vi "GeoData.vi"() -> ()   [LabVIEW 2017] (continued)
29826\t45011\tElko\tSC\tBarnwell County\tH1\n29915\t45013\tDaufuskie island\tSC\tBeaufort County\tH1\n29907\t45013\tBeaufort\tSC\tBeaufort County\tH1\n29910\t45013\tBluffton\tSC\tBeaufort County\tH1\n29909\t45013\tOkatie\tSC\tBeaufort County\tH1\n29906\t45013\tBeaufort\tSC\tBeaufort County\tH1\n29920\t45013\tSaint helena island\tSC\tBeaufort County\tH1\n29925\t45013\tHilton head island\tSC\tBeaufort County\tH1\n29936\t45013\tRidgeland\tSC\tBeaufort County\tH1\n29935\t45013\tPort royal\tSC\tBeaufort County\tH1\n29904\t45013\tBeaufort\tSC\tBeaufort County\tH1\n29926\t45013\tHilton head island\tSC\tBeaufort County\tH1\n29940\t45013\tSeabrook\tSC\tBeaufort County\tH1\n29945\t45013\tYemassee\tSC\tBeaufort County\tH1\n29902\t45013\tBeaufort\tSC\tBeaufort County\tH1\n29903\t45013\tBeaufort\tSC\tBeaufort County\tH1\n29901\t45013\tBeaufort\tSC\tBeaufort County\tH1\n29931\t45013\tLobeco\tSC\tBeaufort County\tH1\n29905\t45013\tParris island\tSC\tBeaufort County\tH1\n29928\t45013\tHilton head island\tSC\tBeaufort County\tH1\n29938\t45013\tHilton head island\tSC\tBeaufort County\tH1\n29941\t45013\tSheldon\tSC\tBeaufort County\tH1\n29431\t45015\tBonneau\tSC\tBerkeley County\tH1\n29456\t45015\tLadson\tSC\tBerkeley County\tH1\n29461\t45015\tMoncks corner\tSC\tBerkeley County\tH1\n29466\t45015\tMount pleasant\tSC\tBerkeley County\tH1\n29469\t45015\tPinopolis\tSC\tBerkeley County\tH1\n29059\t45015\tHolly hill\tSC\tBerkeley County\tH1\n29472\t45015\tRidgeville\tSC\tBerkeley County\tH1\n29406\t45015\tCharleston\tSC\tBerkeley County\tH1\n29492\t45015\tCharleston\tSC\tBerkeley County\tH1\n29453\t45015\tJamestown\tSC\tBerkeley County\tH1\n29445\t45015\tGoose creek\tSC\tBerkeley County\tH1\n29468\t45015\tPineville\tSC\tBerkeley County\tH1\n29450\t45015\tHuger\tSC\tBerkeley County\tH1\n29410\t45015\tHanahan\tSC\tBerkeley County\tH1\n29483\t45015\tSummerville\tSC\tBerkeley County\tH1\n29436\t45015\tCross\tSC\tBerkeley County\tH1\n29486\t45015\tSummerville\tSC\tBerkeley County\tH1\n29434\t45015\tCordesville\tSC\tBerkeley County\tH1\n29479\t45015\tSaint stephen\tSC\tBerkeley County\tH1\n29476\t45015\tRussellville\tSC\tBerkeley County\tH1\n29118\t45017\tOrangeburg\tSC\tCalhoun County\tH1\n29053\t45017\tGaston\tSC\tCalhoun County\tH1\n29135\t45017\tSaint matthews\tSC\tCalhoun County\tH1\n29030\t45017\tCameron\tSC\tCalhoun County\tH1\n29047\t45017\tElloree\tSC\tCalhoun County\tH1\n29160\t45017\tSwansea\tSC\tCalhoun County\tH1\n29112\t45017\tNorth\tSC\tCalhoun County\tH1\n29455\t45019\tJohns island\tSC\tCharleston County\tH1\n29449\t45019\tHollywood\tSC\tCharleston County\tH1\n29424\t45019\tCharleston\tSC\tCharleston County\tH1\n29456\t45019\tLadson\tSC\tCharleston County\tH1\n29466\t45019\tMount pleasant\tSC\tCharleston County\tH1\n29465\t45019\tMount pleasant\tSC\tCharleston County\tH1\n29417\t45019\tCharleston\tSC\tCharleston County\tH1\n29412\t45019\tCharleston\tSC\tCharleston County\tH1\n29401\t45019\tCharleston\tSC\tCharleston County\tH1\n29419\t45019\tNorth charleston\tSC\tCharleston County\tH1\n29413\t45019\tCharleston\tSC\tCharleston County\tH1\n29439\t45019\tFolly beach\tSC\tCharleston County\tH1\n29406\t45019\tCharleston\tSC\tCharleston County\tH1\n29438\t45019\tEdisto island\tSC\tCharleston County\tH1\n29429\t45019\tAwendaw\tSC\tCharleston County\tH1\n29464\t45019\tMount pleasant\tSC\tCharleston County\tH1\n29485\t45019\tSummerville\tSC\tCharleston County\tH1\n29470\t45019\tRavenel\tSC\tCharleston County\tH1\n29453\t45019\tJamestown\tSC\tCharleston County\tH1\n29409\t45019\tCharleston\tSC\tCharleston County\tH1\n29451\t45019\tIsle of palms\tSC\tCharleston County\tH1\n29450\t45019\tHuger\tSC\tCharleston County\tH1\n29482\t45019\tSullivans island\tSC\tCharleston County\tH1\n29416\t45019\tCharleston\tSC\tCharleston County\tH1\n29426\t45019\tAdams run\tSC\tCharleston County\tH1\n29403\t45019\tCharleston\tSC\tCharleston County\tH1\n29407\t45019\tCharleston\tSC\tCharleston County\tH1\n29405\t45019\tNorth charleston\tSC\tCharleston County\tH1\n29410\t45019\tHanahan\tSC\tCharleston County\tH1\n29422\t45019\tCharleston\tSC\tCharleston County\tH1\n29483\t45019\tSummerville\tSC\tCharleston County\tH1\n29415\t45019\tNorth charleston\tSC\tCharleston County\tH1\n29425\t45019\tCharleston\tSC\tCharleston County\tH1\n29404\t45019\tCharleston afb\tSC\tCharleston County\tH1\n29418\t45019\tNorth charleston\tSC\tCharleston County\tH1\n29420\t45019\tNorth charleston\tSC\tCharleston County\tH1\n29414\t45019\tCharleston\tSC\tCharleston County\tH1\n29487\t45019\tWadmalaw island\tSC\tCharleston County\tH1\n29423\t45019\tCharleston\tSC\tCharleston County\tH1\n29402\t45019\tCharleston\tSC\tCharleston County\tH1\n29458\t45019\tMc clellanville\tSC\tCharleston County\tH1\n29457\t45019\tJohns island\tSC\tCharleston County\tH1\n29702\t45021\tBlacksburg\tSC\tCherokee County\tH1\n29306\t45021\tSpartanburg\tSC\tCherokee County\tH1\n29323\t45021\tChesnee\tSC\tCherokee County\tH1\n29341\t45021\tGaffney\tSC\tCherokee County\tH1\n29330\t45021\tCowpens\tSC\tCherokee County\tH1\n29372\t45021\tPacolet\tSC\tCherokee County\tH1\n29340\t45021\tGaffney\tSC\tCherokee County\tH1\n29307\t45021\tSpartanburg\tSC\tCherokee County\tH1\n29743\t45021\tSmyrna\tSC\tCherokee County\tH1\n29714\t45023\tFort lawn\tSC\tChester County\tH1\n29031\t45023\tCarlisle\tSC\tChester County\tH1\n29742\t45023\tSharon\tSC\tChester County\tH1\n29706\t45023\tChester\tSC\tChester County\tH1\n29014\t45023\tBlackstock\tSC\tChester County\tH1\n29704\t45023\tCatawba\tSC\tChester County\tH1\n29730\t45023\tRock hill\tSC\tChester County\tH1\n29712\t45023\tEdgemoor\tSC\tChester County\tH1\n29729\t45023\tRichburg\tSC\tChester County\tH1\n29055\t45023\tGreat falls\tSC\tChester County\tH1\n29720\t45025\tLancaster\tSC\tChesterfield County\tH1\n29584\t45025\tPatrick\tSC\tChesterfield County\tH1\n29741\t45025\tRuby\tSC\tChesterfield County\tH1\n29520\t45025\tCheraw\tSC\tChesterfield County\tH1\n29727\t45025\tMount croghan\tSC\tChesterfield County\tH1\n29101\t45025\tMc bee\tSC\tChesterfield County\tH1\n29718\t45025\tJefferson\tSC\tChesterfield County\tH1\n29009\t45025\tBethune\tSC\tChesterfield County\tH1\n29550\t45025\tHartsville\tSC\tChesterfield County\tH1\n29593\t45025\tSociety hill\tSC\tChesterfield County\tH1\n29728\t45025\tPageland\tSC\tChesterfield County\tH1\n29709\t45025\tChesterfield\tSC\tChesterfield County\tH1\n29111\t45027\tNew zion\tSC\tClarendon County\tH1\n29056\t45027\tGreeleyville\tSC\tClarendon County\tH1\n29162\t45027\tTurbeville\tSC\tClarendon County\tH1\n29102\t45027\tManning\tSC\tClarendon County\tH1\n29148\t45027\tSummerton\tSC\tClarendon County\tH1\n29518\t45027\tCades\tSC\tClarendon County\tH1\n29041\t45027\tDavis station\tSC\tClarendon County\tH1\n29051\t45027\tGable\tSC\tClarendon County\tH1\n29114\t45027\tOlanta\tSC\tClarendon County\tH1\n29001\t45027\tAlcolu\tSC\tClarendon County\tH1\n29125\t45027\tPinewood\tSC\tClarendon County\tH1\n29560\t45027\tLake city\tSC\tClarendon County\tH1\n29474\t45029\tRound o\tSC\tColleton County\tH1\n29475\t45029\tRuffin\tSC\tColleton County\tH1\n29472\t45029\tRidgeville\tSC\tColleton County\tH1\n29438\t45029\tEdisto island\tSC\tColleton County\tH1\n29446\t45029\tGreen pond\tSC\tColleton County\tH1\n29945\t45029\tYemassee\tSC\tColleton County\tH1\n29081\t45029\tEhrhardt\tSC\tColleton County\tH1\n29481\t45029\tSmoaks\tSC\tColleton County\tH1\n29929\t45029\tIslandton\tSC\tColleton County\tH1\n29452\t45029\tJacksonboro\tSC\tColleton County\tH1\n29082\t45029\tLodge\tSC\tColleton County\tH1\n29435\t45029\tCottageville\tSC\tColleton County\tH1\n29432\t45029\tBranchville\tSC\tColleton County\tH1\n29488\t45029\tWalterboro\tSC\tColleton County\tH1\n29493\t45029\tWilliams\tSC\tColleton County\tH1\n29501\t45031\tFlorence\tSC\tDarlington County\tH1\n29540\t45031\tDarlington\tSC\tDarlington County\tH1\n29101\t45031\tMc bee\tSC\tDarlington County\tH1\n29551\t45031\tHartsville\tSC\tDarlington County\tH1\n29069\t45031\tLamar\tSC\tDarlington County\tH1\n29161\t45031\tTimmonsville\tSC\tDarlington County\tH1\n29550\t45031\tHartsville\tSC\tDarlington County\tH1\n29593\t45031\tSociety hill\tSC\tDarlington County\tH1\n29079\t45031\tLydia\tSC\tDarlington County\tH1\n29506\t45031\tFlorence\tSC\tDarlington County\tH1\n29532\t45031\tDarlington\tSC\tDarlington County\tH1\n29574\t45033\tMullins\tSC\tDillon County\tH1\n29536\t45033\tDillon\tSC\tDillon County\tH1\n29565\t45033\tLatta\tSC\tDillon County\tH1\n29567\t45033\tLittle rock\tSC\tDillon County\tH1\n29563\t45033\tLake view\tSC\tDillon County\tH1\n29581\t45033\tNichols\tSC\tDillon County\tH1\n29592\t45033\tSellers\tSC\tDillon County\tH1\n29547\t45033\tHamer\tSC\tDillon County\tH1\n29525\t45033\tClio\tSC\tDillon County\tH1\n29543\t45033\tFork\tSC\tDillon County\tH1\n29571\t45033\tMarion\tSC\tDillon County\tH1\n29437\t45035\tDorchester\tSC\tDorchester County\tH1\n29456\t45035\tLadson\tSC\tDorchester County\tH1\n29484\t45035\tSummerville\tSC\tDorchester County\tH1\n29472\t45035\tRidgeville\tSC\tDorchester County\tH1\n29471\t45035\tReevesville\tSC\tDorchester County\tH1\n29485\t45035\tSummerville\tSC\tDorchester County\tH1\n29470\t45035\tRavenel\tSC\tDorchester County\tH1\n29426\t45035\tAdams run\tSC\tDorchester County\tH1\n29483\t45035\tSummerville\tSC\tDorchester County\tH1\n29418\t45035\tNorth charleston\tSC\tDorchester County\tH1\n29420\t45035\tNorth charleston\tSC\tDorchester County\tH1\n29414\t45035\tCharleston\tSC\tDorchester County\tH1\n29432\t45035\tBranchville\tSC\tDorchester County\tH1\n29477\t45035\tSaint george\tSC\tDorchester County\tH1\n29447\t45035\tGrover\tSC\tDorchester County\tH1\n29018\t45035\tBowman\tSC\tDorchester County\tH1\n29448\t45035\tHarleyville\tSC\tDorchester County\tH1\n29841\t45037\tNorth augusta\tSC\tEdgefield County\tH1\n29129\t45037\tRidge spring\tSC\tEdgefield County\tH1\n29138\t45037\tSaluda\tSC\tEdgefield County\tH1\n29824\t45037\tEdgefield\tSC\tEdgefield County\tH1\n29838\t45037\tModoc\tSC\tEdgefield County\tH1\n29847\t45037\tTrenton\tSC\tEdgefield County\tH1\n29821\t45037\tClarks hill\tSC\tEdgefield County\tH1\n29860\t45037\tNorth augusta\tSC\tEdgefield County\tH1\n29835\t45037\tMc cormick\tSC\tEdgefield County\tH1\n29845\t45037\tPlum branch\tSC\tEdgefield County\tH1\n29832\t45037\tJohnston\tSC\tEdgefield County\tH1\n29065\t45039\tJenkinsville\tSC\tFairfield County\tH1\n29015\t45039\tBlair\tSC\tFairfield County\tH1\n29031\t45039\tCarlisle\tSC\tFairfield County\tH1\n29045\t45039\tElgin\tSC\tFairfield County\tH1\n29180\t45039\tWinnsboro\tSC\tFairfield County\tH1\n29014\t45039\tBlackstock\tSC\tFairfield County\tH1\n29016\t45039\tBlythewood\tSC\tFairfield County\tH1\n29132\t45039\tRion\tSC\tFairfield County\tH1\n29130\t45039\tRidgeway\tSC\tFairfield County\tH1\n29055\t45039\tGreat falls\tSC\tFairfield County\tH1\n29162\t45041\tTurbeville\tSC\tFlorence County\tH1\n29501\t45041\tFlorence\tSC\tFlorence County\tH1\n29541\t45041\tEffingham\tSC\tFlorence County\tH1\n29555\t45041\tJohnsonville\tSC\tFlorence County\tH1\n29502\t45041\tFlorence\tSC\tFlorence County\tH1\n29505\t45041\tFlorence\tSC\tFlorence County\tH1\n29554\t45041\tHemingway\tSC\tFlorence County\tH1\n29504\t45041\tFlorence\tSC\tFlorence County\tH1\n29591\t45041\tScranton\tSC\tFlorence County\tH1\n29114\t45041\tOlanta\tSC\tFlorence County\tH1\n29161\t45041\tTimmonsville\tSC\tFlorence County\tH1\n29503\t45041\tFlorence\tSC\tFlorence County\tH1\n29506\t45041\tFlorence\tSC\tFlorence County\tH1\n29532\t45041\tDarlington\tSC\tFlorence County\tH1\n29530\t45041\tCoward\tSC\tFlorence County\tH1\n29560\t45041\tLake city\tSC\tFlorence County\tH1\n29583\t45041\tPamplico\tSC\tFlorence County\tH1\n29585\t45043\tPawleys island\tSC\tGeorgetown County\tH1\n29442\t45043\tGeorgetown\tSC\tGeorgetown County\tH1\n29554\t45043\tHemingway\tSC\tGeorgetown County\tH1\n29576\t45043\tMurrells inlet\tSC\tGeorgetown County\tH1\n29440\t45043\tGeorgetown\tSC\tGeorgetown County\tH1\n29510\t45043\tAndrews\tSC\tGeorgetown County\tH1\n29609\t45045\tGreenville\tSC\tGreenville County\tH1\n29627\t45045\tBelton\tSC\tGreenville County\tH1\n29688\t45045\tTigerville\tSC\tGreenville County\tH1\n29356\t45045\tLandrum\tSC\tGreenville County\tH1\n29611\t45045\tGreenville\tSC\tGreenville County\tH1\n29687\t45045\tTaylors\tSC\tGreenville County\tH1\n29636\t45045\tConestee\tSC\tGreenville County\tH1\n29322\t45045\tCampobello\tSC\tGreenville County\tH1\n29607\t45045\tGreenville\tSC\tGreenville County\tH1\n29606\t45045\tGreenville\tSC\tGreenville County\tH1\n29662\t45045\tMauldin\tSC\tGreenville County\tH1\n29602\t45045\tGreenville\tSC\tGreenville County\tH1\n29610\t45045\tGreenville\tSC\tGreenville County\tH1\n29669\t45045\tPelzer\tSC\tGreenville County\tH1\n29680\t45045\tSimpsonville\tSC\tGreenville County\tH1\n29605\t45045\tGreenville\tSC\tGreenville County\tH1\n29644\t45045\tFountain inn\tSC\tGreenville County\tH1\n29661\t45045\tMarietta\tSC\tGreenville County\tH1\n29652\t45045\tGreer\tSC\tGreenville County\tH1\n29681\t45045\tSimpsonville\tSC\tGreenville County\tH1\n29690\t45045\tTravelers rest\tSC\tGreenville County\tH1\n29608\t45045\tGreenville\tSC\tGreenville County\tH1\n29604\t45045\tGreenville\tSC\tGreenville County\tH1\n29683\t45045\tSlater\tSC\tGreenville County\tH1\n29614\t45045\tGreenville\tSC\tGreenville County\tH1\n29613\t45045\tGreenville\tSC\tGreenville County\tH1\n29615\t45045\tGreenville\tSC\tGreenville County\tH1\n29617\t45045\tGreenville\tSC\tGreenville County\tH1\n29654\t45045\tHonea path\tSC\tGreenville County\tH1\n29616\t45045\tGreenville\tSC\tGreenville County\tH1\n29601\t45045\tGreenville\tSC\tGreenville County\tH1\n29673\t45045\tPiedmont\tSC\tGreenville County\tH1\n29635\t45045\tCleveland\tSC\tGreenville County\tH1\n29651\t45045\tGreer\tSC\tGreenville County\tH1\n29650\t45045\tGreer\tSC\tGreenville County\tH1\n29603\t45045\tGreenville\tSC\tGreenville County\tH1\n29612\t45045\tGreenville\tSC\tGreenville County\tH1\n29649\t45047\tGreenwood\tSC\tGreenwood County\tH1\n29647\t45047\tGreenwood\tSC\tGreenwood County\tH1\n29638\t45047\tDonalds\tSC\tGreenwood County\tH1\n29648\t45047\tGreenwood\tSC\tGreenwood County\tH1\n29138\t45047\tSaluda\tSC\tGreenwood County\tH1\n29646\t45047\tGreenwood\tSC\tGreenwood County\tH1\n29653\t45047\tHodges\tSC\tGreenwood County\tH1\n29819\t45047\tBradley\tSC\tGreenwood County\tH1\n29848\t45047\tTroy\tSC\tGreenwood County\tH1\n29695\t45047\tHodges\tSC\tGreenwood County\tH1\n29692\t45047\tWare shoals\tSC\tGreenwood County\tH1\n29666\t45047\tNinety six\tSC\tGreenwood County\tH1\n29922\t45049\tGarnett\tSC\tHampton County\tH1\n29827\t45049\tFairfax\tSC\tHampton County\tH1\n29932\t45049\tLuray\tSC\tHampton County\tH1\n29923\t45049\tGifford\tSC\tHampton County\tH1\n29939\t45049\tScotia\tSC\tHampton County\tH1\n29934\t45049\tPineland\tSC\tHampton County\tH1\n29921\t45049\tFurman\tSC\tHampton County\tH1\n29911\t45049\tBrunson\tSC\tHampton County\tH1\n29944\t45049\tVarnville\tSC\tHampton County\tH1\n29924\t45049\tHampton\tSC\tHampton County\tH1\n29945\t45049\tYemassee\tSC\tHampton County\tH1\n29918\t45049\tEstill\tSC\tHampton County\tH1\n29933\t45049\tMiley\tSC\tHampton County\tH1\n29916\t45049\tEarly branch\tSC\tHampton County\tH1\n29569\t45051\tLoris\tSC\tHorry County\tH1\n29568\t45051\tLongs\tSC\tHorry County\tH1\n29598\t45051\tNorth myrtle beach\tSC\tHorry County\tH1\n29544\t45051\tGalivants ferry\tSC\tHorry County\tH1\n29588\t45051\tMyrtle beach\tSC\tHorry County\tH1\n29587\t45051\tMyrtle beach\tSC\tHorry County\tH1\n29511\t45051\tAynor\tSC\tHorry County\tH1\n29526\t45051\tConway\tSC\tHorry County\tH1\n29545\t45051\tGreen sea\tSC\tHorry County\tH1\n29566\t45051\tLittle river\tSC\tHorry County\tH1\n29576\t45051\tMurrells inlet\tSC\tHorry County\tH1\n29579\t45051\tMyrtle beach\tSC\tHorry County\tH1\n29581\t45051\tNichols\tSC\tHorry County\tH1\n29577\t45051\tMyrtle beach\tSC\tHorry County\tH1\n29575\t45051\tMyrtle beach\tSC\tHorry County\tH1\n29528\t45051\tConway\tSC\tHorry County\tH1\n29597\t45051\tNorth myrtle beach\tSC\tHorry County\tH1\n29527\t45051\tConway\tSC\tHorry County\tH1\n29572\t45051\tMyrtle beach\tSC\tHorry County\tH1\n29582\t45051\tNorth myrtle beach\tSC\tHorry County\tH1\n29578\t45051\tMyrtle beach\tSC\tHorry County\tH1\n29922\t45053\tGarnett\tSC\tJasper County\tH1\n29943\t45053\tTillman\tSC\tJasper County\tH1\n29909\t45053\tOkatie\tSC\tJasper County\tH1\n29934\t45053\tPineland\tSC\tJasper County\tH1\n29936\t45053\tRidgeland\tSC\tJasper County\tH1\n29944\t45053\tVarnville\tSC\tJasper County\tH1\n29945\t45053\tYemassee\tSC\tJasper County\tH1\n29912\t45053\tCoosawhatchie\tSC\tJasper County\tH1\n29916\t45053\tEarly branch\tSC\tJasper County\tH1\n29927\t45053\tHardeeville\tSC\tJasper County\tH1\n29010\t45055\tBishopville\tSC\tKershaw County\tH1\n29074\t45055\tLiberty hill\tSC\tKershaw County\tH1\n29032\t45055\tCassatt\tSC\tKershaw County\tH1\n29020\t45055\tCamden\tSC\tKershaw County\tH1\n29021\t45055\tCamden\tSC\tKershaw County\tH1\n29045\t45055\tElgin\tSC\tKershaw County\tH1\n29128\t45055\tRembert\tSC\tKershaw County\tH1\n29078\t45055\tLugoff\tSC\tKershaw County\tH1\n29175\t45055\tWestville\tSC\tKershaw County\tH1\n29718\t45055\tJefferson\tSC\tKershaw County\tH1\n29009\t45055\tBethune\tSC\tKershaw County\tH1\n29058\t45055\tHeath springs\tSC\tKershaw County\tH1\n29067\t45055\tKershaw\tSC\tKershaw County\tH1\n29130\t45055\tRidgeway\tSC\tKershaw County\tH1\n29720\t45057\tLancaster\tSC\tLancaster County\tH1\n29721\t45057\tLancaster\tSC\tLancaster County\tH1\n29744\t45057\tVan wyck\tSC\tLancaster County\tH1\n29707\t45057\tFort mill\tSC\tLancaster County\tH1\n29718\t45057\tJefferson\tSC\tLancaster County\tH1\n29058\t45057\tHeath springs\tSC\tLancaster County\tH1\n29067\t45057\tKershaw\tSC\tLancaster County\tH1\n29325\t45059\tClinton\tSC\tLaurens County\tH1\n29360\t45059\tLaurens\tSC\tLaurens County\tH1\n29178\t45059\tWhitmire\tSC\tLaurens County\tH1\n29037\t45059\tChappells\tSC\tLaurens County\tH1\n29388\t45059\tWoodruff\tSC\tLaurens County\tH1\n29644\t45059\tFountain inn\tSC\tLaurens County\tH1\n29681\t45059\tSimpsonville\tSC\tLaurens County\tH1\n29351\t45059\tJoanna\tSC\tLaurens County\tH1\n29384\t45059\tWaterloo\tSC\tLaurens County\tH1\n29654\t45059\tHonea path\tSC\tLaurens County\tH1\n29370\t45059\tMountville\tSC\tLaurens County\tH1\n29332\t45059\tCross hill\tSC\tLaurens County\tH1\n29335\t45059\tEnoree\tSC\tLaurens County\tH1\n29355\t45059\tKinards\tSC\tLaurens County\tH1\n29645\t45059\tGray court\tSC\tLaurens County\tH1\n29692\t45059\tWare shoals\tSC\tLaurens County\tH1\n29010\t45061\tBishopville\tSC\tLee County\tH1\n29032\t45061\tCassatt\tSC\tLee County\tH1\n29020\t45061\tCamden\tSC\tLee County\tH1\n29046\t45061\tElliott\tSC\tLee County\tH1\n29128\t45061\tRembert\tSC\tLee County\tH1\n29080\t45061\tLynchburg\tSC\tLee County\tH1\n29009\t45061\tBethune\tSC\tLee County\tH1\n29040\t45061\tDalzell\tSC\tLee County\tH1\n29104\t45061\tMayesville\tSC\tLee County\tH1\n29069\t45061\tLamar\tSC\tLee County\tH1\n29153\t45061\tSumter\tSC\tLee County\tH1\n29550\t45061\tHartsville\tSC\tLee County\tH1\n29054\t45063\tGilbert\tSC\tLexington County\tH1\n29170\t45063\tWest columbia\tSC\tLexington County\tH1\n29169\t45063\tWest columbia\tSC\tLexington County\tH1\n29171\t45063\tWest columbia\tSC\tLexington County\tH1\n29212\t45063\tColumbia\tSC\tLexington County\tH1\n29071\t45063\tLexington\tSC\tLexington County\tH1\n29053\t45063\tGaston\tSC\tLexington County\tH1\n29033\t45063\tCayce\tSC\tLexington County\tH1\n29210\t45063\tColumbia\tSC\tLexington County\tH1\n29072\t45063\tLexington\tSC\tLexington County\tH1\n29172\t45063\tWest columbia\tSC\tLexington County\tH1\n29006\t45063\tBatesburg\tSC\tLexington County\tH1\n29070\t45063\tLeesville\tSC\tLexington County\tH1\n29073\t45063\tLexington\tSC\tLexington County\tH1\n29075\t45063\tLittle mountain\tSC\tLexington County\tH1\n29063\t45063\tIrmo\tSC\tLexington County\tH1\n29160\t45063\tSwansea\tSC\tLexington County\tH1\n29214\t45063\tColumbia\tSC\tLexington County\tH1\n29036\t45063\tChapin\tSC\tLexington County\tH1\n29112\t45063\tNorth\tSC\tLexington County\tH1\n29123\t45063\tPelion\tSC\tLexington County\tH1\n29620\t45065\tAbbeville\tSC\tMcCormick County\tH1\n29844\t45065\tParksville\tSC\tMcCormick County\tH1\n29838\t45065\tModoc\tSC\tMcCormick County\tH1\n29899\t45065\tMc cormick\tSC\tMcCormick County\tH1\n29628\t45065\tCalhoun falls\tSC\tMcCormick County\tH1\n29819\t45065\tBradley\tSC\tMcCormick County\tH1\n29848\t45065\tTroy\tSC\tMcCormick County\tH1\n29821\t45065\tClarks hill\tSC\tMcCormick County\tH1\n29835\t45065\tMc cormick\tSC\tMcCormick County\tH1\n29840\t45065\tMount carmel\tSC\tMcCormick County\tH1\n29845\t45065\tPlum branch\tSC\tMcCormick County\tH1\n29574\t45067\tMullins\tSC\tMarion County\tH1\n29589\t45067\tRains\tSC\tMarion County\tH1\n29546\t45067\tGresham\tSC\tMarion County\tH1\n29565\t45067\tLatta\tSC\tMarion County\tH1\n29519\t45067\tCentenary\tSC\tMarion County\tH1\n29581\t45067\tNichols\tSC\tMarion County\tH1\n29592\t45067\tSellers\tSC\tMarion County\tH1\n29571\t45067\tMarion\tSC\tMarion County\tH1\n29570\t45069\tMc coll\tSC\tMarlboro County\tH1\n29565\t45069\tLatta\tSC\tMarlboro County\tH1\n29596\t45069\tWallace\tSC\tMarlboro County\tH1\n29516\t45069\tBlenheim\tSC\tMarlboro County\tH1\n29594\t45069\tTatum\tSC\tMarlboro County\tH1\n29512\t45069\tBennettsville\tSC\tMarlboro County\tH1\n29525\t45069\tClio\tSC\tMarlboro County\tH1\n29145\t45071\tSilverstreet\tSC\tNewberry County\tH1\n29126\t45071\tPomaria\tSC\tNewberry County\tH1\n29178\t45071\tWhitmire\tSC\tNewberry County\tH1\n29037\t45071\tChappells\tSC\tNewberry County\tH1\n29108\t45071\tNewberry\tSC\tNewberry County\tH1\n29122\t45071\tPeak\tSC\tNewberry County\tH1\n29075\t45071\tLittle mountain\tSC\tNewberry County\tH1\n29332\t45071\tCross hill\tSC\tNewberry County\tH1\n29355\t45071\tKinards\tSC\tNewberry County\tH1\n29036\t45071\tChapin\tSC\tNewberry County\tH1\n29127\t45071\tProsperity\tSC\tNewberry County\tH1\n29676\t45073\tSalem\tSC\tOconee County\tH1\n29696\t45073\tWest union\tSC\tOconee County\tH1\n29643\t45073\tFair play\tSC\tOconee County\tH1\n29664\t45073\tMountain rest\tSC\tOconee County\tH1\n29672\t45073\tSeneca\tSC\tOconee County\tH1\n29658\t45073\tLong creek\tSC\tOconee County\tH1\n29689\t45073\tTownville\tSC\tOconee County\tH1\n29678\t45073\tSeneca\tSC\tOconee County\tH1\n29679\t45073\tSeneca\tSC\tOconee County\tH1\n29686\t45073\tTamassee\tSC\tOconee County\tH1\n29693\t45073\tWestminster\tSC\tOconee County\tH1\n29691\t45073\tWalhalla\tSC\tOconee County\tH1\n29665\t45073\tNewry\tSC\tOconee County\tH1\n29675\t45073\tRichland\tSC\tOconee County\tH1\n29118\t45075\tOrangeburg\tSC\tOrangeburg County\tH1\n29133\t45075\tRowesville\tSC\tOrangeburg County\tH1\n29163\t45075\tVance\tSC\tOrangeburg County\tH1\n29059\t45075\tHolly hill\tSC\tOrangeburg County\tH1\n29107\t45075\tNeeses\tSC\tOrangeburg County\tH1\n29135\t45075\tSaint matthews\tSC\tOrangeburg County\tH1\n29146\t45075\tSpringfield\tSC\tOrangeburg County\tH1\n29142\t45075\tSantee\tSC\tOrangeburg County\tH1\n29038\t45075\tCope\tSC\tOrangeburg County\tH1\n29039\t45075\tCordova\tSC\tOrangeburg County\tH1\n29115\t45075\tOrangeburg\tSC\tOrangeburg County\tH1\n29471\t45075\tReevesville\tSC\tOrangeburg County\tH1\n29113\t45075\tNorway\tSC\tOrangeburg County\tH1\n29030\t45075\tCameron\tSC\tOrangeburg County\tH1\n29137\t45075\tSalley\tSC\tOrangeburg County\tH1\n29048\t45075\tEutawville\tSC\tOrangeburg County\tH1\n29117\t45075\tOrangeburg\tSC\tOrangeburg County\tH1\n29047\t45075\tElloree\tSC\tOrangeburg County\tH1\n29160\t45075\tSwansea\tSC\tOrangeburg County\tH1\n29436\t45075\tCross\tSC\tOrangeburg County\tH1\n29432\t45075\tBranchville\tSC\tOrangeburg County\tH1\n29477\t45075\tSaint george\tSC\tOrangeburg County\tH1\n29018\t45075\tBowman\tSC\tOrangeburg County\tH1\n29112\t45075\tNorth\tSC\tOrangeburg County\tH1\n29116\t45075\tOrangeburg\tSC\tOrangeburg County\tH1\n29671\t45077\tPickens\tSC\tPickens County\tH1\n29682\t45077\tSix mile\tSC\tPickens County\tH1\n29611\t45077\tGreenville\tSC\tPickens County\tH1\n29633\t45077\tClemson\tSC\tPickens County\tH1\n29630\t45077\tCentral\tSC\tPickens County\tH1\n29661\t45077\tMarietta\tSC\tPickens County\tH1\n29670\t45077\tPendleton\tSC\tPickens County\tH1\n29631\t45077\tClemson\tSC\tPickens County\tH1\n29642\t45077\tEasley\tSC\tPickens County\tH1\n29657\t45077\tLiberty\tSC\tPickens County\tH1\n29667\t45077\tNorris\tSC\tPickens County\tH1\n29685\t45077\tSunset\tSC\tPickens County\tH1\n29635\t45077\tCleveland\tSC\tPickens County\tH1\n29632\t45077\tClemson\tSC\tPickens County\tH1\n29640\t45077\tEasley\tSC\tPickens County\tH1\n29641\t45077\tEasley\tSC\tPickens County\tH1\n29634\t45077\tClemson\tSC\tPickens County\tH1\n29202\t45079\tColumbia\tSC\tRichland County\tH1\n29205\t45079\tColumbia\tSC\tRichland County\tH1\n29240\t45079\tColumbia\tSC\tRichland County\tH1\n29215\t45079\tColumbia\tSC\tRichland County\tH1\n29226\t45079\tColumbia\tSC\tRichland County\tH1\n29204\t45079\tColumbia\tSC\tRichland County\tH1\n29209\t45079\tColumbia\tSC\tRichland County\tH1\n29212\t45079\tColumbia\tSC\tRichland County\tH1\n29229\t45079\tColumbia\tSC\tRichland County\tH1\n29223\t45079\tColumbia\tSC\tRichland County\tH1\n29208\t45079\tColumbia\tSC\tRichland County\tH1\n29260\t45079\tColumbia\tSC\tRichland County\tH1\n29177\t45079\tWhite rock\tSC\tRichland County\tH1\n29219\t45079\tColumbia\tSC\tRichland County\tH1\n29225\t45079\tColumbia\tSC\tRichland County\tH1\n29201\t45079\tColumbia\tSC\tRichland County\tH1\n29210\t45079\tColumbia\tSC\tRichland County\tH1\n29250\t45079\tColumbia\tSC\tRichland County\tH1\n29217\t45079\tColumbia\tSC\tRichland County\tH1\n29147\t45079\tState park\tSC\tRichland County\tH1\n29045\t45079\tElgin\tSC\tRichland County\tH1\n29180\t45079\tWinnsboro\tSC\tRichland County\tH1\n29218\t45079\tColumbia\tSC\tRichland County\tH1\n29220\t45079\tColumbia\tSC\tRichland County\tH1\n29292\t45079\tColumbia\tSC\tRichland County\tH1\n29078\t45079\tLugoff\tSC\tRichland County\tH1\n29207\t45079\tColumbia\tSC\tRichland County\tH1\n29002\t45079\tBallentine\tSC\tRichland County\tH1\n29222\t45079\tColumbia\tSC\tRichland County\tH1\n29016\t45079\tBlythewood\tSC\tRichland County\tH1\n29044\t45079\tEastover\tSC\tRichland County\tH1\n29211\t45079\tColumbia\tSC\tRichland County\tH1\n29075\t45079\tLittle mountain\tSC\tRichland County\tH1\n29224\t45079\tColumbia\tSC\tRichland County\tH1\n29230\t45079\tColumbia\tSC\tRichland County\tH1\n29063\t45079\tIrmo\tSC\tRichland County\tH1\n29206\t45079\tColumbia\tSC\tRichland County\tH1\n29221\t45079\tColumbia\tSC\tRichland County\tH1\n29214\t45079\tColumbia\tSC\tRichland County\tH1\n29036\t45079\tChapin\tSC\tRichland County\tH1\n29061\t45079\tHopkins\tSC\tRichland County\tH1\n29052\t45079\tGadsden\tSC\tRichland County\tH1\n29130\t45079\tRidgeway\tSC\tRichland County\tH1\n29203\t45079\tColumbia\tSC\tRichland County\tH1\n29290\t45079\tColumbia\tSC\tRichland County\tH1\n29227\t45079\tColumbia\tSC\tRichland County\tH1\n29216\t45079\tColumbia\tSC\tRichland County\tH1\n29129\t45081\tRidge spring\tSC\tSaluda County\tH1\n29138\t45081\tSaluda\tSC\tSaluda County\tH1\n29824\t45081\tEdgefield\tSC\tSaluda County\tH1\n29166\t45081\tWard\tSC\tSaluda County\tH1\n29006\t45081\tBatesburg\tSC\tSaluda County\tH1\n29037\t45081\tChappells\tSC\tSaluda County\tH1\n29848\t45081\tTroy\tSC\tSaluda County\tH1\n29070\t45081\tLeesville\tSC\tSaluda County\tH1\n29832\t45081\tJohnston\tSC\tSaluda County\tH1\n29105\t45081\tMonetta\tSC\tSaluda County\tH1\n29127\t45081\tProsperity\tSC\tSaluda County\tH1\n29666\t45081\tNinety six\tSC\tSaluda County\tH1\n29306\t45083\tSpartanburg\tSC\tSpartanburg County\tH1\n29369\t45083\tMoore\tSC\tSpartanburg County\tH1\n29304\t45083\tSpartanburg\tSC\tSpartanburg County\tH1\n29338\t45083\tFingerville\tSC\tSpartanburg County\tH1\n29316\t45083\tBoiling springs\tSC\tSpartanburg County\tH1\n29323\t45083\tChesnee\tSC\tSpartanburg County\tH1\n29349\t45083\tInman\tSC\tSpartanburg County\tH1\n29356\t45083\tLandrum\tSC\tSpartanburg County\tH1\n29324\t45083\tClifton\tSC\tSpartanburg County\tH1\n29377\t45083\tStartex\tSC\tSpartanburg County\tH1\n29322\t45083\tCampobello\tSC\tSpartanburg County\tH1\n29330\t45083\tCowpens\tSC\tSpartanburg County\tH1\n29376\t45083\tRoebuck\tSC\tSpartanburg County\tH1\n29372\t45083\tPacolet\tSC\tSpartanburg County\tH1\n29336\t45083\tFairforest\tSC\tSpartanburg County\tH1\n29378\t45083\tUna\tSC\tSpartanburg County\tH1\n29319\t45083\tSpartanburg\tSC\tSpartanburg County\tH1\n29388\t45083\tWoodruff\tSC\tSpartanburg County\tH1\n29375\t45083\tReidville\tSC\tSpartanburg County\tH1\n29305\t45083\tSpartanburg\tSC\tSpartanburg County\tH1\n29302\t45083\tSpartanburg\tSC\tSpartanburg County\tH1\n29303\t45083\tSpartanburg\tSC\tSpartanburg County\tH1\n29307\t45083\tSpartanburg\tSC\tSpartanburg County\tH1\n29374\t45083\tPauline\tSC\tSpartanburg County\tH1\n29346\t45083\tGlendale\tSC\tSpartanburg County\tH1\n29320\t45083\tArcadia\tSC\tSpartanburg County\tH1\n29329\t45083\tConverse\tSC\tSpartanburg County\tH1\n29301\t45083\tSpartanburg\tSC\tSpartanburg County\tH1\n29335\t45083\tEnoree\tSC\tSpartanburg County\tH1\n29334\t45083\tDuncan\tSC\tSpartanburg County\tH1\n29365\t45083\tLyman\tSC\tSpartanburg County\tH1\n29385\t45083\tWellford\tSC\tSpartanburg County\tH1\n29333\t45083\tDrayton\tSC\tSpartanburg County\tH1\n29368\t45083\tMayo\tSC\tSpartanburg County\tH1\n29386\t45083\tWhite stone\tSC\tSpartanburg County\tH1\n29331\t45083\tCross anchor\tSC\tSpartanburg County\tH1\n29348\t45083\tGramling\tSC\tSpartanburg County\tH1\n29651\t45083\tGreer\tSC\tSpartanburg County\tH1\n29650\t45083\tGreer\tSC\tSpartanburg County\tH1\n29373\t45083\tPacolet mills\tSC\tSpartanburg County\tH1\n29168\t45085\tWedgefield\tSC\tSumter County\tH1\n29150\t45085\tSumter\tSC\tSumter County\tH1\n29162\t45085\tTurbeville\tSC\tSumter County\tH1\n29102\t45085\tManning\tSC\tSumter County\tH1\n29128\t45085\tRembert\tSC\tSumter County\tH1\n29154\t45085\tSumter\tSC\tSumter County\tH1\n29080\t45085\tLynchburg\tSC\tSumter County\tH1\n29152\t45085\tShaw afb\tSC\tSumter County\tH1\n29040\t45085\tDalzell\tSC\tSumter County\tH1\n29051\t45085\tGable\tSC\tSumter County\tH1\n29104\t45085\tMayesville\tSC\tSumter County\tH1\n29114\t45085\tOlanta\tSC\tSumter County\tH1\n29153\t45085\tSumter\tSC\tSumter County\tH1\n29151\t45085\tSumter\tSC\tSumter County\tH1\n29001\t45085\tAlcolu\tSC\tSumter County\tH1\n29125\t45085\tPinewood\tSC\tSumter County\tH1\n29062\t45085\tHoratio\tSC\tSumter County\tH1\n29031\t45087\tCarlisle\tSC\tUnion County\tH1\n29178\t45087\tWhitmire\tSC\tUnion County\tH1\n29372\t45087\tPacolet\tSC\tUnion County\tH1\n29364\t45087\tLockhart\tSC\tUnion County\tH1\n29379\t45087\tUnion\tSC\tUnion County\tH1\n29321\t45087\tBuffalo\tSC\tUnion County\tH1\n29374\t45087\tPauline\tSC\tUnion County\tH1\n29335\t45087\tEnoree\tSC\tUnion County\tH1\n29353\t45087\tJonesville\tSC\tUnion County\tH1\n29395\t45087\tJonesville\tSC\tUnion County\tH1\n29111\t45089\tNew zion\tSC\tWilliamsburg County\tH1\n29556\t45089\tKingstree\tSC\tWilliamsburg County\tH1\n29580\t45089\tNesmith\tSC\tWilliamsburg County\tH1\n29056\t45089\tGreeleyville\tSC\tWilliamsburg County\tH1\n29555\t45089\tJohnsonville\tSC\tWilliamsburg County\tH1\n29554\t45089\tHemingway\tSC\tWilliamsburg County\tH1\n29518\t45089\tCades\tSC\tWilliamsburg County\tH1\n29440\t45089\tGeorgetown\tSC\tWilliamsburg County\tH1\n29510\t45089\tAndrews\tSC\tWilliamsburg County\tH1\n29564\t45089\tLane\tSC\tWilliamsburg County\tH1\n29590\t45089\tSalters\tSC\tWilliamsburg County\tH1\n29560\t45089\tLake city\tSC\tWilliamsburg County\tH1\n29702\t45091\tBlacksburg\tSC\tYork County\tH1\n29745\t45091\tYork\tSC\tYork County\tH1\n29726\t45091\tMc connells\tSC\tYork County\tH1\n29732\t45091\tRock hill\tSC\tYork County\tH1\n29742\t45091\tSharon\tSC\tYork County\tH1\n29703\t45091\tBowling green\tSC\tYork County\tH1\n29706\t45091\tChester\tSC\tYork County\tH1\n29707\t45091\tFort mill\tSC\tYork County\tH1\n29710\t45091\tClover\tSC\tYork County\tH1\n29717\t45091\tHickory grove\tSC\tYork County\tH1\n29731\t45091\tRock hill\tSC\tYork County\tH1\n29716\t45091\tFort mill\tSC\tYork County\tH1\n29734\t45091\tRock hill\tSC\tYork County\tH1\n29733\t45091\tRock hill\tSC\tYork County\tH1\n29708\t45091\tFort mill\tSC\tYork County\tH1\n29704\t45091\tCatawba\tSC\tYork County\tH1\n29715\t45091\tFort mill\tSC\tYork County\tH1\n29730\t45091\tRock hill\tSC\tYork County\tH1\n29712\t45091\tEdgemoor\tSC\tYork County\tH1\n29743\t45091\tSmyrna\tSC\tYork County\tH1\n57369\t46003\tPlatte\tSD\tAurora County\tH1\n57328\t46003\tCorsica\tSD\tAurora County\tH1\n57363\t46003\tMount vernon\tSD\tAurora County\tH1\n57385\t46003\tWoonsocket\tSD\tAurora County\tH1\n57382\t46003\tWessington springs\tSD\tAurora County\tH1\n57375\t46003\tStickney\tSD\tAurora County\tH1\n57359\t46003\tLetcher\tSD\tAurora County\tH1\n57383\t46003\tWhite lake\tSD\tAurora County\tH1\n57368\t46003\tPlankinton\tSD\tAurora County\tH1\n57312\t46005\tAlpena\tSD\tBeadle County\tH1\n57324\t46005\tCavour\tSD\tBeadle County\tH1\n57381\t46005\tWessington\tSD\tBeadle County\tH1\n57384\t46005\tWolsey\tSD\tBeadle County\tH1\n57314\t46005\tArtesian\tSD\tBeadle County\tH1\n57322\t46005\tCarpenter\tSD\tBeadle County\tH1\n57382\t46005\tWessington springs\tSD\tBeadle County\tH1\n57386\t46005\tYale\tSD\tBeadle County\tH1\n57350\t46005\tHuron\tSD\tBeadle County\tH1\n57348\t46005\tHitchcock\tSD\tBeadle County\tH1\n57353\t46005\tIroquois\tSD\tBeadle County\tH1\n57379\t46005\tVirgil\tSD\tBeadle County\tH1\n57399\t46005\tHuron\tSD\tBeadle County\tH1\n57574\t46007\tTuthill\tSD\tBennett County\tH1\n57551\t46007\tMartin\tSD\tBennett County\tH1\n57566\t46007\tParmelee\tSD\tBennett County\tH1\n57716\t46007\tBatesland\tSD\tBennett County\tH1\n57714\t46007\tAllen\tSD\tBennett County\tH1\n57560\t46007\tNorris\tSD\tBennett County\tH1\n57063\t46009\tTabor\tSD\tBon Homme County\tH1\n57315\t46009\tAvon\tSD\tBon Homme County\tH1\n57059\t46009\tScotland\tSD\tBon Homme County\tH1\n57040\t46009\tLesterville\tSD\tBon Homme County\tH1\n57062\t46009\tSpringfield\tSD\tBon Homme County\tH1\n57066\t46009\tTyndall\tSD\tBon Homme County\tH1\n57376\t46009\tTripp\tSD\tBon Homme County\tH1\n57234\t46011\tEstelline\tSD\tBrookings County\tH1\n57220\t46011\tBruce\tSD\tBrookings County\tH1\n57268\t46011\tToronto\tSD\tBrookings County\tH1\n57276\t46011\tWhite\tSD\tBrookings County\tH1\n57026\t46011\tElkton\tSD\tBrookings County\tH1\n57002\t46011\tAurora\tSD\tBrookings County\tH1\n57212\t46011\tArlington\tSD\tBrookings County\tH1\n57006\t46011\tBrookings\tSD\tBrookings County\tH1\n57213\t46011\tAstoria\tSD\tBrookings County\tH1\n57007\t46011\tBrookings\tSD\tBrookings County\tH1\n57071\t46011\tVolga\tSD\tBrookings County\tH1\n57061\t46011\tSinai\tSD\tBrookings County\tH1\n57451\t46013\tIpswich\tSD\tBrown County\tH1\n57433\t46013\tColumbia\tSD\tBrown County\tH1\n57460\t46013\tMansfield\tSD\tBrown County\tH1\n57449\t46013\tHoughton\tSD\tBrown County\tH1\n57481\t46013\tWestport\tSD\tBrown County\tH1\n57434\t46013\tConde\tSD\tBrown County\tH1\n57426\t46013\tBarnard\tSD\tBrown County\tH1\n57446\t46013\tHecla\tSD\tBrown County\tH1\n57441\t46013\tFrederick\tSD\tBrown County\tH1\n57432\t46013\tClaremont\tSD\tBrown County\tH1\n57402\t46013\tAberdeen\tSD\tBrown County\tH1\n57422\t46013\tAndover\tSD\tBrown County\tH1\n57401\t46013\tAberdeen\tSD\tBrown County\tH1\n57445\t46013\tGroton\tSD\tBrown County\tH1\n57439\t46013\tFerney\tSD\tBrown County\tH1\n57427\t46013\tBath\tSD\tBrown County\tH1\n57461\t46013\tMellette\tSD\tBrown County\tH1\n57474\t46013\tStratford\tSD\tBrown County\tH1\n57479\t46013\tWarner\tSD\tBrown County\tH1\n57370\t46015\tPukwana\tSD\tBrule County\tH1\n57369\t46015\tPlatte\tSD\tBrule County\tH1\n57325\t46015\tChamberlain\tSD\tBrule County\tH1\n57523\t46015\tBurke\tSD\tBrule County\tH1\n57355\t46015\tKimball\tSD\tBrule County\tH1\n57383\t46015\tWhite lake\tSD\tBrule County\tH1\n57370\t46017\tPukwana\tSD\tBuffalo County\tH1\n57339\t46017\tFort thompson\tSD\tBuffalo County\tH1\n57362\t46017\tMiller\tSD\tBuffalo County\tH1\n57325\t46017\tChamberlain\tSD\tBuffalo County\tH1\n57341\t46017\tGann valley\tSD\tBuffalo County\tH1\n57760\t46019\tNewell\tSD\tButte County\tH1\n57779\t46019\tSaint onge\tSD\tButte County\tH1\n57788\t46019\tVale\tSD\tButte County\tH1\n57783\t46019\tSpearfish\tSD\tButte County\tH1\n57717\t46019\tBelle fourche\tSD\tButte County\tH1\n57758\t46019\tMud butte\tSD\tButte County\tH1\n57762\t46019\tNisland\tSD\tButte County\tH1\n57437\t46021\tEureka\tSD\tCampbell County\tH1\n57648\t46021\tPollock\tSD\tCampbell County\tH1\n57631\t46021\tGlenham\tSD\tCampbell County\tH1\n57601\t46021\tMobridge\tSD\tCampbell County\tH1\n57472\t46021\tSelby\tSD\tCampbell County\tH1\n57646\t46021\tMound city\tSD\tCampbell County\tH1\n57452\t46021\tJava\tSD\tCampbell County\tH1\n57632\t46021\tHerreid\tSD\tCampbell County\tH1\n57313\t46023\tArmour\tSD\tCharles Mix County\tH1\n57369\t46023\tPlatte\tSD\tCharles Mix County\tH1\n57315\t46023\tAvon\tSD\tCharles Mix County\tH1\n57367\t46023\tPickstown\tSD\tCharles Mix County\tH1\n57329\t46023\tDante\tSD\tCharles Mix County\tH1\n57361\t46023\tMarty\tSD\tCharles Mix County\tH1\n57330\t46023\tDelmont\tSD\tCharles Mix County\tH1\n57356\t46023\tLake andes\tSD\tCharles Mix County\tH1\n57376\t46023\tTripp\tSD\tCharles Mix County\tH1\n57380\t46023\tWagner\tSD\tCharles Mix County\tH1\n57342\t46023\tGeddes\tSD\tCharles Mix County\tH1\n57434\t46025\tConde\tSD\tClark County\tH1\n57221\t46025\tBryant\tSD\tClark County\tH1\n57271\t46025\tVienna\tSD\tClark County\tH1\n57272\t46025\tWallace\tSD\tClark County\tH1\n57274\t46025\tWebster\tSD\tClark County\tH1\n57278\t46025\tWillow lake\tSD\tClark County\tH1\n57322\t46025\tCarpenter\tSD\tClark County\tH1\n57243\t46025\tHenry\tSD\tClark County\tH1\n57225\t46025\tClark\tSD\tClark County\tH1\n57217\t46025\tBradley\tSD\tClark County\tH1\n57353\t46025\tIroquois\tSD\tClark County\tH1\n57236\t46025\tGarden city\tSD\tClark County\tH1\n57258\t46025\tRaymond\tSD\tClark County\tH1\n57069\t46027\tVermillion\tSD\tClay County\tH1\n57073\t46027\tWakonda\tSD\tClay County\tH1\n57014\t46027\tCenterville\tSD\tClay County\tH1\n57010\t46027\tBurbank\tSD\tClay County\tH1\n57072\t46027\tVolin\tSD\tClay County\tH1\n57037\t46027\tIrene\tSD\tClay County\tH1\n57031\t46027\tGayville\tSD\tClay County\tH1\n57004\t46027\tBeresford\tSD\tClay County\tH1\n57235\t46029\tFlorence\tSD\tCodington County\tH1\n57238\t46029\tGoodwin\tSD\tCodington County\tH1\n57263\t46029\tSouth shore\tSD\tCodington County\tH1\n57242\t46029\tHazel\tSD\tCodington County\tH1\n57272\t46029\tWallace\tSD\tCodington County\tH1\n57265\t46029\tStrandburg\tSD\tCodington County\tH1\n57201\t46029\tWatertown\tSD\tCodington County\tH1\n57243\t46029\tHenry\tSD\tCodington County\tH1\n57217\t46029\tBradley\tSD\tCodington County\tH1\n57264\t46029\tStockholm\tSD\tCodington County\tH1\n57256\t46029\tOrtley\tSD\tCodington County\tH1\n57245\t46029\tKranzburg\tSD\tCodington County\tH1\n57642\t46031\tMc laughlin\tSD\tCorson County\tH1\n57657\t46031\tTrail city\tSD\tCorson County\tH1\n57645\t46031\tMorristown\tSD\tCorson County\tH1\n57641\t46031\tMc intosh\tSD\tCorson County\tH1\n57659\t46031\tWalker\tSD\tCorson County\tH1\n57658\t46031\tWakpala\tSD\tCorson County\tH1\n57638\t46031\tLemmon\tSD\tCorson County\tH1\n57644\t46031\tMeadow\tSD\tCorson County\tH1\n57660\t46031\tWatauga\tSD\tCorson County\tH1\n57621\t46031\tBullhead\tSD\tCorson County\tH1\n57634\t46031\tKeldron\tSD\tCorson County\tH1\n57639\t46031\tLittle eagle\tSD\tCorson County\tH1\n57738\t46033\tFairburn\tSD\tCuster County\tH1\n57722\t46033\tBuffalo gap\tSD\tCuster County\tH1\n57747\t46033\tHot springs\tSD\tCuster County\tH1\n57744\t46033\tHermosa\tSD\tCuster County\tH1\n57735\t46033\tEdgemont\tSD\tCuster County\tH1\n57730\t46033\tCuster\tSD\tCuster County\tH1\n57751\t46033\tKeystone\tSD\tCuster County\tH1\n57773\t46033\tPringle\tSD\tCuster County\tH1\n57328\t46035\tCorsica\tSD\tDavison County\tH1\n57363\t46035\tMount vernon\tSD\tDavison County\tH1\n57334\t46035\tEthan\tSD\tDavison County\tH1\n57301\t46035\tMitchell\tSD\tDavison County\tH1\n57331\t46035\tDimock\tSD\tDavison County\tH1\n57375\t46035\tStickney\tSD\tDavison County\tH1\n57359\t46035\tLetcher\tSD\t
